vi "Multiple Setpoint Setup.vi"(9 "Number of Setpoints":u8, 10 "Multiple Setpoints?":bool, 11 "SCADA in":refnum<class "SCADA.lvclass">) -> (3 "SCADA out":refnum<class "SCADA.lvclass">)   [LabVIEW 2015, in "SCADA Core.lvlib" / "SCADA.lvclass"]
uses:
  SCADA.lvclass
  SCADA.lvclass/SCADA.ctl
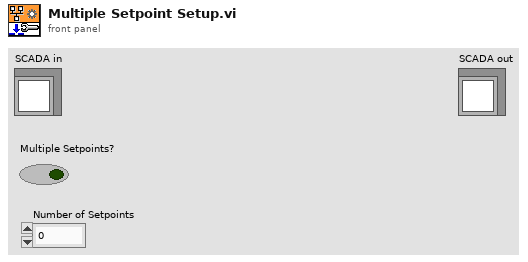
[diagram p1: front panel]
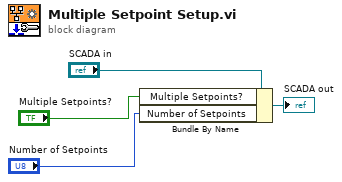
[diagram p0: block diagram]
diagram:
  n1 = Bundle By Name(cluster="SCADA in", "Multiple Setpoints?"="Multiple Setpoints?", "Number of Setpoints"="Number of Setpoints") -> (→"SCADA out":refnum<class "SCADA.lvclass">)
